vi "isJilSmartDevice.vi"(11 "device":string) -> (3 "x != y?":bool)   [LabVIEW 2010]
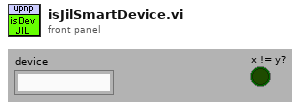
[diagram p1: front panel]
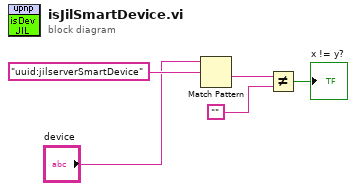
[diagram p0: block diagram]
diagram:
  n1 = Match Pattern(string="device", regular expression="uuid:jilserverSmartDevice") -> (after substring=w5:string)  [unwired: 4 out]
  n2 = Not Equal?(x=w5, y="") -> (x != y?=→"x != y?":bool)
